vi "Initialize Device Core.vi"(8 "error in (no error)":errorcluster, 9 "Reset (F)":bool, 10 "Resource Name":string, 11 "BNT_DAQmx-MCSV-DOPWM in":refnum<class "BNT_DAQmx-MCSV-DOPWM.lvclass">) -> (0 "error out":errorcluster, 3 "BNT_DAQmx-MCSV-DOPWM out":refnum<class "BNT_DAQmx-MCSV-DOPWM.lvclass">)   [LabVIEW 2021, in "BNT_DAQmx.lvlib" / "BNT_DAQmx-MCSV-DOPWM.lvclass"]
doc: "Initialize device driver."
uses:
  BNT_DAQmx-MCSV-DOPWM.lvclass
  C:/Users/Holger/Documents/LVP/BNT/EQCR/Packages/BNT_DAQmx/BNT_DAQmx-MCSV/BNT_DAQmx-MCSV.lvclass
  BNT_DAQmx-MCSV/BNT_DAQmx-MCSV.lvclass/BNT_DAQmx-MCSV.ctl
  BNT_DAQmx-MCSV-DOPWM.lvclass/BNT_DAQmx-MCSV-DOPWM.ctl
  BNT_DAQmx-MCSV/BNT_DAQmx-MCSV.lvclass
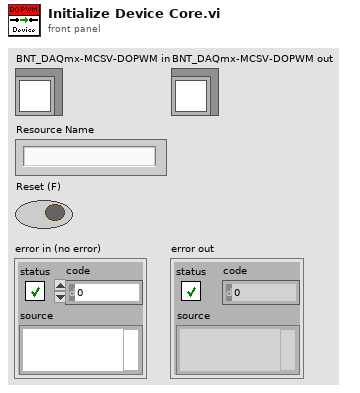
[diagram p1: front panel]
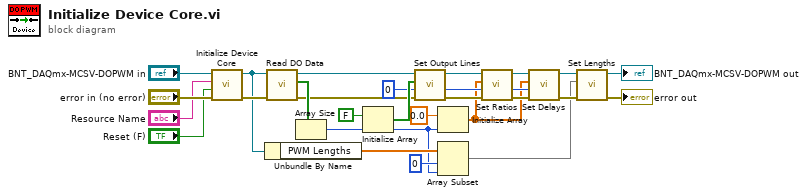
[diagram p0: block diagram]
diagram:
  w11 = 0 ("Start Index")
  n1 = call-parent "Initialize Device Core.vi"("error in (no error)"="error in (no error)", "Reset (F)"="Reset (F)", "Resource Name"="Resource Name", "BNT_DAQmx-MCSV in"="BNT_DAQmx-MCSV-DOPWM in") -> ("error out"=w17:errorcluster, "BNT_DAQmx-MCSV out"=w9:refnum<class "BNT_DAQmx-MCSV-DOPWM.lvclass">)  [unwired: 6 in]
  n2 = Unbundle By Name(w9) -> ("PWM Lengths"=w8:dbl[unit][])
  n3 = call "Read DO Data.vi"("error in (no error)"=w17, "BNT_DAQmx-MCSV in"=w9) -> ("error out"=w18:errorcluster, "DO Data"=w20:bool[], "BNT_DAQmx-MCSV out"=w19:refnum<class "BNT_DAQmx-MCSV-DOPWM.lvclass">)  [unwired: 7 in]
  n4 = Array Size(array=w20) -> (size(s)=w6:i32)
  n5 = Initialize Array(FALSE, w6) -> (w21:bool[])
  n6 = call "Set Output Lines.vi"("Error In"=w18, "Start Index"=w11, "DO Lines"=w21, "BNT_DAQmx-MCSV in"=w19) -> ("Error Out"=w15:errorcluster, "BNT_DAQmx-MCSV out"=w16:refnum<class "BNT_DAQmx-MCSV-DOPWM.lvclass">)  [unwired: 6 in]
  n7 = Initialize Array(0.0, w6) -> (w10:dbl[])
  n8 = Array Subset(array=w8, index=0, length=w6) -> (w1:dbl[unit][])
  n9 = call "Set Ratios.vi"("error in"=w15, "Start Index"=w11, "PWM Ratios"=w10, "BNT_DAQmx-MCSV-DOPWM in"=w16) -> ("error out"=w13:errorcluster, "BNT_DAQmx-MCSV-DOPWM out"=w14:refnum<class "BNT_DAQmx-MCSV-DOPWM.lvclass">)  [unwired: 6 in]
  n10 = call "Set Delays.vi"("error in"=w13, "Start Index"=w11, "PWM Delays"=w10, "BNT_DAQmx-MCSV-DOPWM in"=w14) -> ("error out"=w3:errorcluster, "BNT_DAQmx-MCSV-DOPWM out"=w5:refnum<class "BNT_DAQmx-MCSV-DOPWM.lvclass">)  [unwired: 6 in]
  n11 = call "Set Lengths.vi"("error in"=w3, "PWM Lengths"=w1, "BNT_DAQmx-MCSV-DOPWM in"=w5) -> ("error out"=→"error out":errorcluster, "BNT_DAQmx-MCSV-DOPWM out"=→"BNT_DAQmx-MCSV-DOPWM out":refnum<class "BNT_DAQmx-MCSV-DOPWM.lvclass">)  [unwired: 7 in]
